vi "DPIDs.Find.vi"(10 "ID":u8, 11 "DPIDs":T1[](array[typedef])) -> (2 "Found":bool, 3 "DPID":T1)   [LabVIEW 2019, in "Diagnostics Addon Engine.lvlib"]
uses:
  Diagnostics Addon Engine.lvlib
  Shared/Types/DPID.ctl
  Shared/Types/DPID.Rate.ctl
  Shared/Diagnostics Addon Shared.lvlib
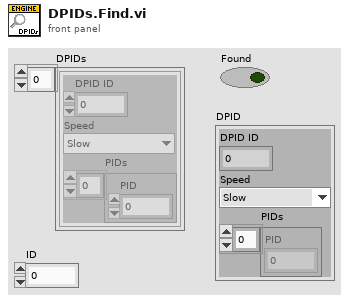
[diagram p1: front panel]
types:
  T1 = typedef "Diagnostics Addon Shared.lvlib/DPID.ctl" = cluster{"DPID ID":u8, "Speed":T2, "PIDs":u16[]}
  T2 = typedef "Diagnostics Addon Shared.lvlib/DPID.Rate.ctl" = enum16{"Slow", "Medium", "Fast"}
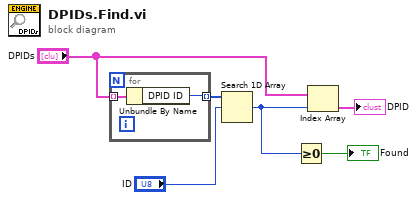
[diagram p0: block diagram]
diagram:
  n1 = for {
    tunnel: "DPIDs" -> [w8] mode=indexing
    tunnel: [w7] -> w1 mode=indexing
    n2 = Unbundle By Name(w8) -> ("DPID ID"=w7:u8)
  }
  n3 = Search 1D Array(1D array=w1, element="ID") -> (index of element=w6:i32)  [unwired: 1 in]
  n4 = Greater Or Equal To 0?(x=w6) -> (x >= 0?=→"Found":bool)
  n5 = Index Array(array="DPIDs", index=w6) -> (element=→"DPID":T1)
